vi "Render.vi"(8 "error in (no error)":errorcluster, 10 "String in":string, 11 "OrderedList in":refnum<class "OrderedList.lvclass">) -> (0 "error out":errorcluster, 2 "String out":string, 3 "OrderedList out":refnum<class "OrderedList.lvclass">)   [LabVIEW 2021, in "LvMarkdown.lvlib" / "OrderedList.lvclass"]
uses:
  OrderedList.lvclass
  OrderedList.lvclass/OrderedList.ctl
  Collection/GetElements.vi
  IRenderable/IRenderable.lvclass
  Collection/Collection.lvclass
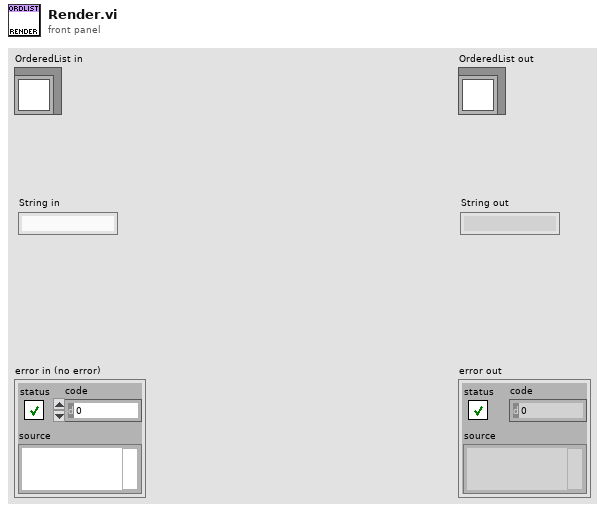
[diagram p1: front panel]
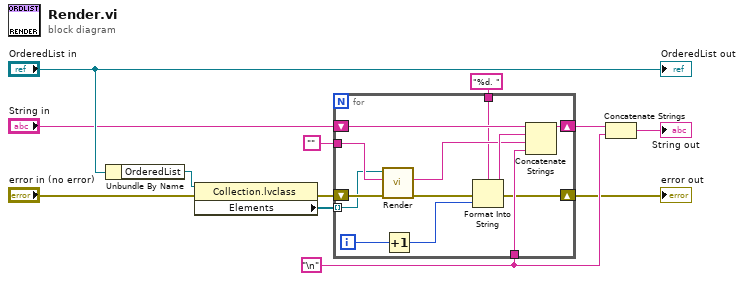
[diagram p0: block diagram]
diagram:
  w8 = "\n"
  n1 = Unbundle By Name("OrderedList in") -> ("OrderedList"=w11:refnum<class "Collection.lvclass">)
  n2 = property class="Collection.lvclass"(reference=w11, error in="error in (no error)") -> (error out=w2:errorcluster, "Elements"=w1:refnum<class "IRenderable.lvclass">[])  [unwired: 1 out]
  n3 = for {
    shift-right: [w24] -> w9
    shift-left: "String in" -> [w25]
    tunnel: w8 -> [w19]
    tunnel: "" -> [w17]
    shift-right: [w15] -> w5
    shift-left: w2 -> [w18]
    tunnel: "%d. " ("format string") -> [w14]
    tunnel: w1 -> [w13] mode=indexing
    i -> [w22]
    n4 = call-dynamic "Render.vi"("error in (no error)"=w18, "String in"=w17, "IRenderable in"=w13) -> ("error out"=w16:errorcluster, "String out"=w20:string)  [unwired: 6 in, 1 out]
    n5 = Increment(x=w22) -> (x+1=w21:i32)
    n6 = Format Into String(format string=w14, error in=w16, w21) -> (resulting string=w23:string, error out=w15:errorcluster)  [unwired: 1 in]
    n7 = Concatenate Strings(w25, w23, w20, w19) -> (w24:string)
  }
  "error out" <- w5
  n8 = Concatenate Strings(w9, w8) -> (→"String out":string)
  "OrderedList out" <- "OrderedList in"
